vi "Get Type.vi"(11 "Boolean in":refnum<class "Boolean.lvclass">) -> (3 "Type":string)   [LabVIEW 2020, in "Boolean.lvclass"]
uses:
  <vilib>/gpm_packages/@cs/data-type-serializer/source/Boolean/Boolean.lvclass
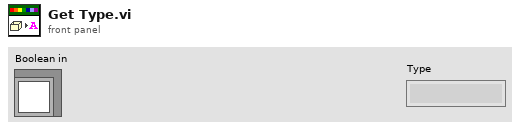
[diagram p1: front panel]
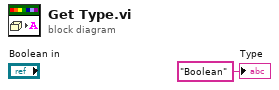
[diagram p0: block diagram]
diagram:
  "Type" <- "Boolean" ("Type")
